vi "Read Configuration Parameters.vi"(8 "error in (no error)":errorcluster, 10 "refnum":T1, 11 "DAQ Configuration in":refnum<class "DAQ Configuration.lvclass">) -> (0 "error out":errorcluster, 2 "refnum out":T1, 3 "DAQ Configuration out":refnum<class "DAQ Configuration.lvclass">)   [LabVIEW 2016, in "Hardware.lvlib" / "DAQ Configuration.lvclass"]
uses:
  DAQ Configuration.lvclass
  <vilib>/Utility/config.llb/Config Data RefNum.ctl
  DAQ Configuration.lvclass/DAQ Configuration.ctl
  HW Config/HW Configuration.lvclass
  <vilib>/Utility/config.llb/NI_LVConfig.lvlib
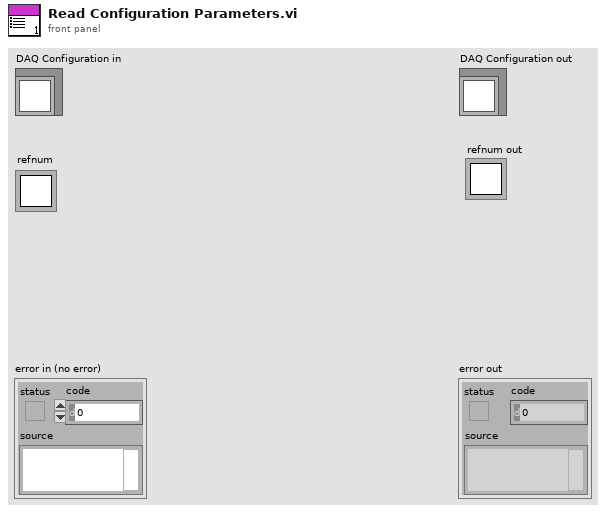
[diagram p1: front panel]
types:
  T1 = typedef "NI_LVConfig.lvlib/Config Data RefNum.ctl" = refnum<k1>
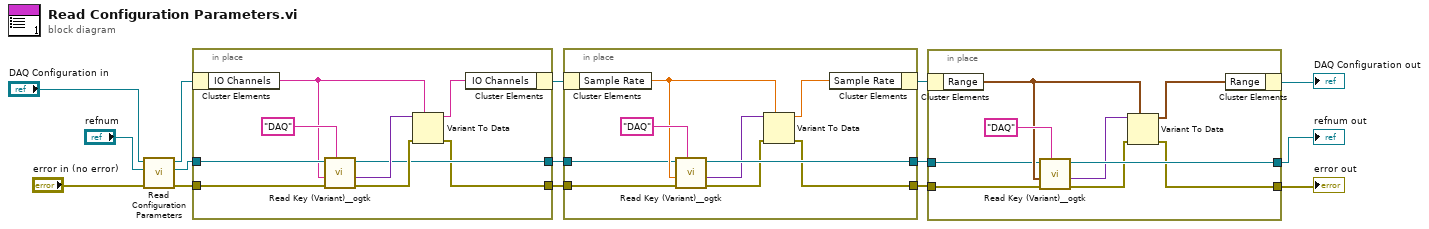
[diagram p0: block diagram]
diagram:
  n1 = call-parent "Read Configuration Parameters.vi"("error in (no error)"="error in (no error)", "refnum"="refnum", "Configuration in"="DAQ Configuration in") -> ("error out"=w7:errorcluster, "refnum out"=w8:T1, "Configuration out"=w9:refnum<class "DAQ Configuration.lvclass">)  [unwired: 6 in]
  n2 = in-place "In Place Element Structure" {
    in-place-border: w8 -> [w22]
    in-place-border: w7 -> [w16]
    in-place-border: [w20] -> w11
    in-place-border: [w19] -> w10
    n3 = in-place-cluster #1(w9) -> ("IO Channels"=w18:string)
    n4 = call <userlib>:"Read Key (Variant)__ogtk.vi"("section"="DAQ", "error in (no error)"=w16, "type"=w18, "refnum"=w22) -> ("error out"=w23:errorcluster, "key-value"=w24:variant, "refnum out"=w20:T1)  [unwired: 4 in, 1 out]
    n5 = Variant To Data(error in=w23, type=w18, Variant=w24) -> (data=w17:string, error out=w19:errorcluster)
    n6 = in-place-cluster #1("IO Channels"=w17) -> (w12:refnum<class "DAQ Configuration.lvclass">)
  }
  n7 = in-place "In Place Element Structure" {
    in-place-border: [w27] -> w6
    in-place-border: [w32] -> w5
    in-place-border: w11 -> [w26]
    in-place-border: w10 -> [w25]
    n8 = in-place-cluster #2(w12) -> ("Sample Rate"=w31:dbl)
    n9 = call <userlib>:"Read Key (Variant)__ogtk.vi"("section"="DAQ", "error in (no error)"=w25, "type"=w31, "refnum"=w26) -> ("error out"=w28:errorcluster, "key-value"=w30:variant, "refnum out"=w32:T1)  [unwired: 4 in, 1 out]
    n10 = Variant To Data(error in=w28, type=w31, Variant=w30) -> (data=w29:dbl, error out=w27:errorcluster)
    n11 = in-place-cluster #2("Sample Rate"=w29) -> (w4:refnum<class "DAQ Configuration.lvclass">)
  }
  n12 = in-place "In Place Element Structure" {
    in-place-border: [w36] -> w1
    in-place-border: [w41] -> w2
    in-place-border: w5 -> [w35]
    in-place-border: w6 -> [w34]
    n13 = in-place-cluster #3(w4) -> ("Range"=w40:cluster{"Ranve (min)":dbl, "Range Max":dbl})
    n14 = call <userlib>:"Read Key (Variant)__ogtk.vi"("section"="DAQ", "error in (no error)"=w34, "type"=w40, "refnum"=w35) -> ("error out"=w37:errorcluster, "key-value"=w39:variant, "refnum out"=w41:T1)  [unwired: 4 in, 1 out]
    n15 = Variant To Data(error in=w37, type=w40, Variant=w39) -> (data=w38:cluster{"Ranve (min)":dbl, "Range Max":dbl}, error out=w36:errorcluster)
    n16 = in-place-cluster #3("Range"=w38) -> (→"DAQ Configuration out":refnum<class "DAQ Configuration.lvclass">)
  }
  "error out" <- w1
  "refnum out" <- w2
